vi "WLAN Rx Test Set Parameters.vi"(8 "error in (no error)":errorcluster, 10 "Parameters":T1={"Standard"=enum."802.11 n HT", "DSSS Data Rate (Mbps)"=enum."1", "OFDM Data Rate (Mbps)"=enum."54", "MCS Index"=7, "N Spatial Streams"=1, "Chains"=[TRUE, FALSE, FALSE, FALSE], "Bandwidth (Hz)"=enum."20 MHz", "Channel"=1, "Power (dBm)"=0.0, "Guard Interval"=enum."SHORT", "FEC Coding"=enum."LDPC", "16 symbols"=TRUE, "Payload Length (bytes)"=1500, "Idle Interval (s)"=0.0001, "External Attenuation (dB)"=[0.0, 0.0, 0.0, 0.0], "RX Measurement Parameters"={"Number of Packets"=1000, "MacAddress"="FF:FF:FF:FF:FF:FF"}} {"Idle Interval (s)" format="%_3p"}, 11 "WLAN Tx Test in":refnum<class "niDTS WLAN Rx Test.lvclass">) -> (0 "error out":errorcluster, 3 "WLAN Tx Test out":refnum<class "niDTS WLAN Rx Test.lvclass">)   [LabVIEW 2015, in "niDTS WLAN.lvlib" / "niDTS WLAN Rx Test.lvclass"]
uses:
  niDTS WLAN Rx Test.lvclass
  Includes/niDTS WLAN Rx Test INC Parameters.ctl
  Includes/niDTS WLAN INC Standard.ctl
  Includes/niDTS WLAN INC DSSS Data Rate.ctl
  Includes/niDTS WLAN INC OFDM Data Rate.ctl
  Includes/niDTS WLAN INC CH BW.ctl
  Includes/niDTS WLAN INC GI.ctl
  Includes/niDTS WLAN INC FEC Coding.ctl
  Includes/niDTS WLAN INC RX Measurement Parameters.ctl
  niDTS WLAN Rx Test.lvclass/niDTS WLAN Rx Test.ctl
  niDTS WLAN.lvlib
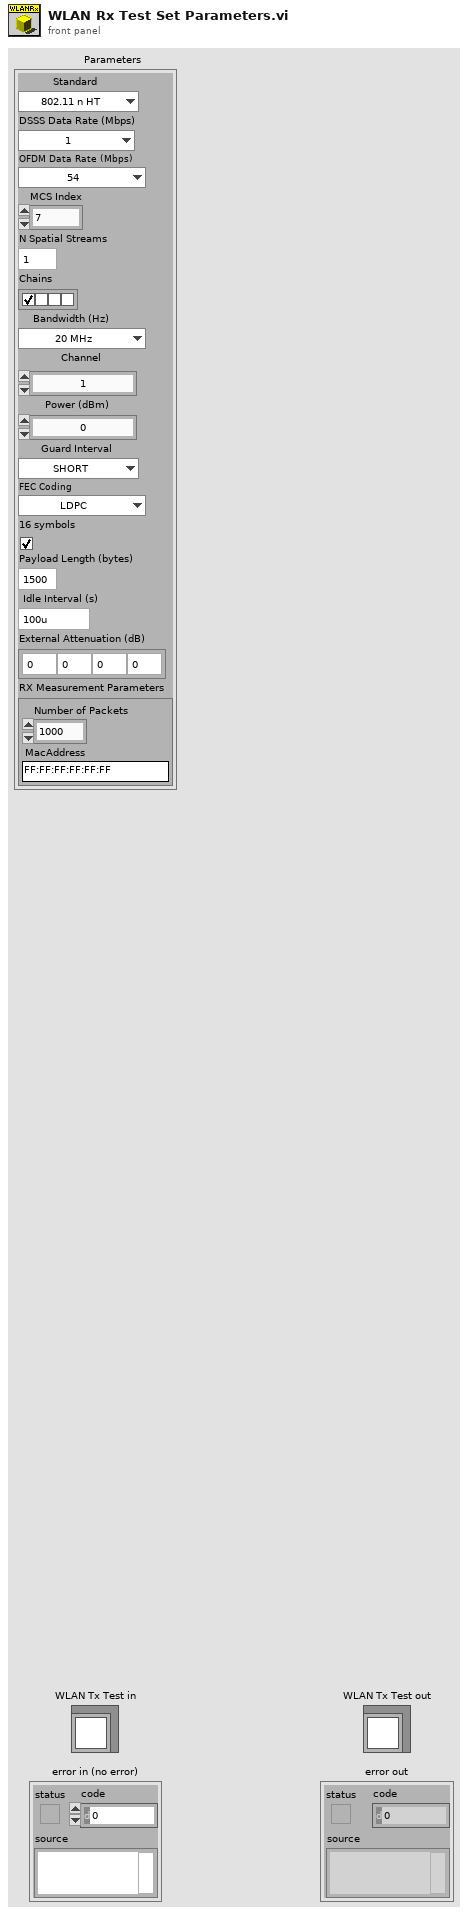
[diagram p1: front panel]
types:
  T1 = typedef "niDTS WLAN.lvlib/niDTS WLAN Rx Test INC Parameters.ctl" = cluster{"Standard":T2, "DSSS Data Rate (Mbps)":T3, "OFDM Data Rate (Mbps)":T4, "MCS Index":i32, "N Spatial Streams":i32, "Chains":bool[], "Bandwidth (Hz)":T5, "Channel":i32, "Power (dBm)":dbl, "Guard Interval":T6, "FEC Coding":T7, "16 symbols":bool, "Payload Length (bytes)":i32, "Idle Interval (s)":dbl, "External Attenuation (dB)":dbl[], "RX Measurement Parameters":T8}
  T2 = typedef "niDTS WLAN.lvlib/niDTS WLAN INC Standard.ctl" = enum16{"802.11 b DSSS", "802.11 a/g OFDM", "802.11 n HT", "802.11 ac VHT"}
  T3 = typedef "niDTS WLAN.lvlib/niDTS WLAN INC DSSS Data Rate.ctl" = enum16{"1", "2", "5.5", "11"}
  T4 = typedef "niDTS WLAN.lvlib/niDTS WLAN INC OFDM Data Rate.ctl" = enum16{"6", "9", "12", "18", "24", "36", "48", "54"}
  T5 = typedef "niDTS WLAN.lvlib/niDTS WLAN INC CH BW.ctl" = enum16{"20 MHz", "40 MHz", "80 MHz", "160 MHz"}
  T6 = typedef "niDTS WLAN.lvlib/niDTS WLAN INC GI.ctl" = enum16{"LONG", "SHORT"}
  T7 = typedef "niDTS WLAN.lvlib/niDTS WLAN INC FEC Coding.ctl" = enum16{"BCC", "LDPC"}
  T8 = typedef "niDTS WLAN.lvlib/niDTS WLAN INC RX Measurement Parameters.ctl" = cluster{"Number of Packets":i32, "MacAddress":string}
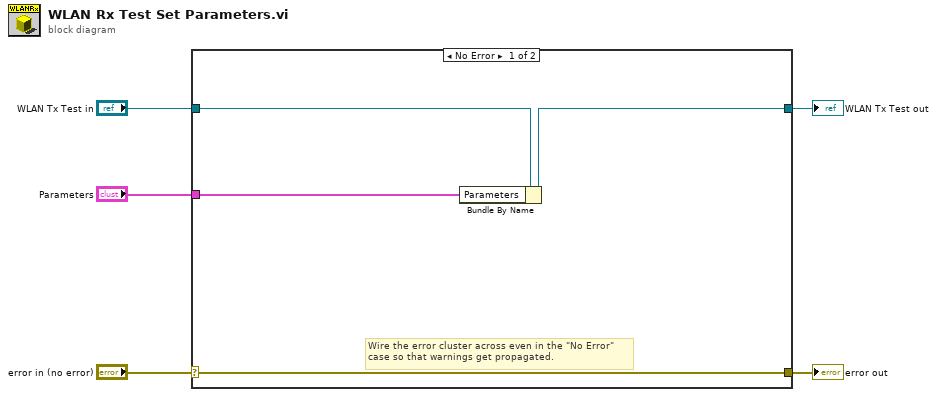
[diagram p0: block diagram]
diagram:
  n1 = case shown="No Error" "error in (no error)" {
    selector: "error in (no error)" -> [w9 w11]
    tunnel: [w9 w11] -> w4
    tunnel: [w7 w10] -> w2
    tunnel: "WLAN Tx Test in" -> [w8 w10]
    tunnel: "Parameters" -> [w6 _]
    frame No Error {
      # "Wire the error cluster across even in the \"No Error\"\ncase so that warnings get propagated."
      n2 = Bundle By Name(cluster=w8, "Parameters"=w6) -> (w7:refnum<class "niDTS WLAN Rx Test.lvclass">)
    }
    frame Error {
    }
  }
  "error out" <- w4
  "WLAN Tx Test out" <- w2
